vi "Round to Value.vi"(1 "Precision":dbl, 2 "Value In":dbl) -> (0 "Rounded":dbl)   [LabVIEW 2010]
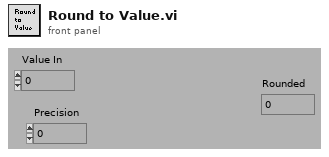
[diagram p1: front panel]
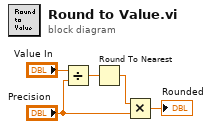
[diagram p0: block diagram]
diagram:
  n1 = Divide(x="Value In", y="Precision") -> (x/y=w4:dbl)
  n2 = Round To Nearest(number=w4) -> (nearest integer value=w3:dbl)
  n3 = Multiply(x=w3, y="Precision") -> (x*y=→"Rounded":dbl)
